vi "Queue Driver.vi"(0 "Enqueue states":string[](array[string]), 2 "Name":string, 11 "Error in":errorcluster, 13 "Queue Operations":T1) -> (4 "Dequeued state":string, 15 "Error out":errorcluster)   [LabVIEW 2020, in "File explorer 2.0.lvlib"]
doc: "This VI is used as a queue driver for simple state machine"
uses:
  File explorer 2.0.lvlib
  Typedefs/Queue operations.ctl
panel:
  # "QUEUE DRIVER"
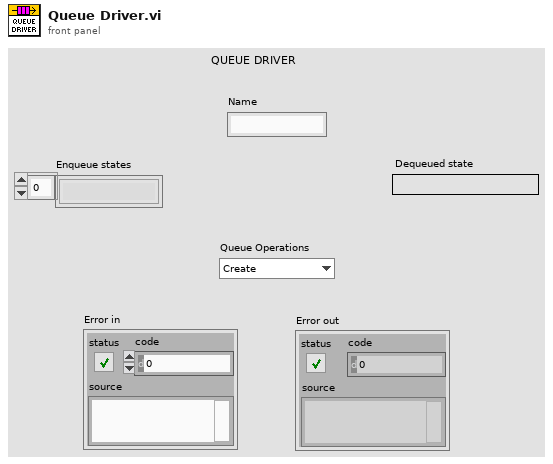
[diagram p1: front panel]
types:
  T1 = typedef "File explorer 2.0.lvlib/Queue operations.ctl" = enum16{"Create", "Enqueue", "Enstack", "Dequeue", "Flush", "Release"}
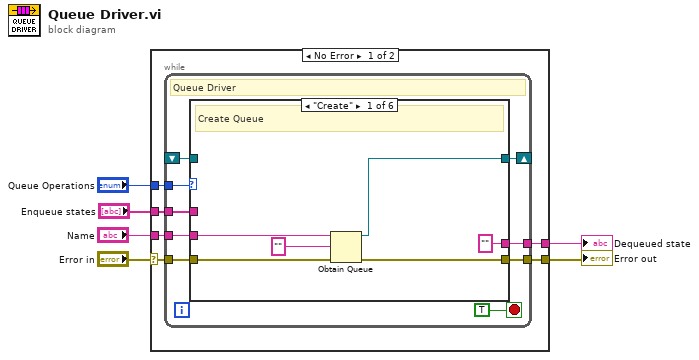
[diagram p0: block diagram]
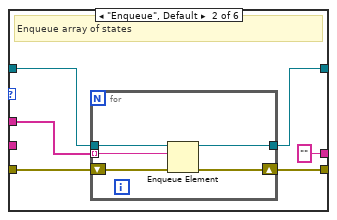
[diagram p2: hidden frame]
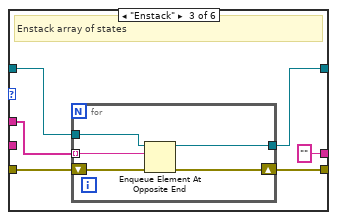
[diagram p3: hidden frame]
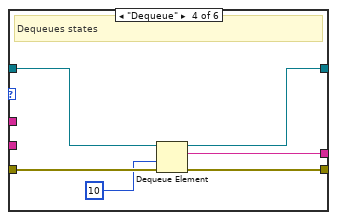
[diagram p4: hidden frame]
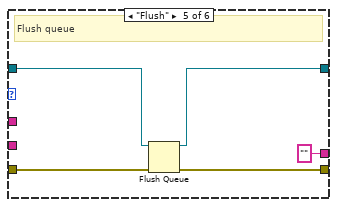
[diagram p5: hidden frame]
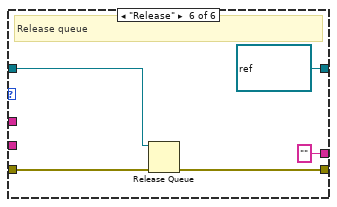
[diagram p6: hidden frame]
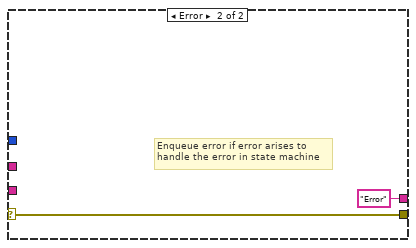
[diagram p7: hidden frame]
diagram:
  n1 = case shown="No Error" "Error in" {
    selector: "Error in" -> [w11 w66]
    tunnel: "Queue Operations" -> [w12 _]
    tunnel: [w10 w66] -> w4
    tunnel: "Name" -> [w9 _]
    tunnel: "Enqueue states" -> [w8 _]
    tunnel: [w7 "Error"] -> w1
    frame No Error {
      n2 = while {
        tunnel: w12 -> [w20]
        tunnel: w11 -> [w19]
        tunnel: [w18] -> w10
        tunnel: w9 -> [w17]
        shift-right: [w15] -> _
        shift-left: _ -> [w14]
        tunnel: w8 -> [w16]
        tunnel: [w13] -> w7
        stop <- TRUE stop-if-true
        # "Queue Driver"
        n3 = case shown="\"Create\"" w20 {
          tunnel: w19 -> [w27 w33 w44 w55 w60 w65]
          tunnel: [w26 w32 w43 w54 w59 w64] -> w18
          tunnel: w17 -> [w25 _ _ _ _ _]
          tunnel: w16 -> [_ w31 w42 _ _ _]
          tunnel: [w24 w30 w40 w52 w57 refnum<queue> refnum ("queue")] -> w15
          tunnel: w14 -> [_ w29 w41 w53 w58 w63]
          tunnel: ["" "" "" w50 "" ""] -> w13
          frame "Create" {
            # "Create Queue"
            n4 = Obtain Queue(name (unnamed)=w25, element data type="" ("Name"), error in (no error)=w27) -> (queue out=w24:refnum<queue>, error out=w26:errorcluster)  [unwired: 2 in, 1 out]
          }
          frame "Enqueue", Default {
            # "Enqueue array of states"
            n5 = for {
              shift-right: [w37] -> w32
              shift-left: w33 -> [w38]
              tunnel: w31 -> [w36] mode=indexing
              tunnel: [w35] -> w30
              tunnel: w29 -> [w34]
              n6 = Enqueue Element(queue=w34, element=w36, error in (no error)=w38) -> (queue out=w35:refnum<queue>, error out=w37:errorcluster)  [unwired: 1 in, 1 out]
            }
          }
          frame "Enstack" {
            # "Enstack array of states"
            n7 = for {
              shift-right: [w48] -> w43
              shift-left: w44 -> [w49]
              tunnel: w42 -> [w47] mode=indexing
              tunnel: w41 -> [w46]
              tunnel: [w45] -> w40
              n8 = Enqueue Element At Opposite End(queue=w46, element=w47, error in (no error)=w49) -> (queue out=w45:refnum<queue>, error out=w48:errorcluster)  [unwired: 1 in, 1 out]
            }
          }
          frame "Dequeue" {
            # "Dequeues states"
            n9 = Dequeue Element(queue=w53, timeout in ms (-1)=10, error in (no error)=w55) -> (queue out=w52:refnum<queue>, element=w50:string, error out=w54:errorcluster)  [unwired: 1 out]
          }
          frame "Flush" {
            # "Flush queue"
            n10 = Flush Queue(queue=w58, error in (no error)=w60) -> (queue out=w57:refnum<queue>, error out=w59:errorcluster)  [unwired: 1 out]
          }
          frame "Release" {
            # "Release queue"
            n11 = Release Queue(queue=w63, error in (no error)=w65) -> (error out=w64:errorcluster)  [unwired: 1 in, 2 out]
          }
        }
      }
    }
    frame Error {
      # "Enqueue error if error arises to\nhandle the error in state machine"
    }
  }
  "Error out" <- w4
  "Dequeued state" <- w1
